vi "Choreo_TrajectoryDifferential_Events.vi"(11 "ChoreoTrajectoryDifferential":T2) -> (3 "events":T1[](array[typedef]))   [LabVIEW 2019, in "ChoreoLib.lvlib"]
doc: "Returns the events in the trajectory.\n\nInputs:\n -- ChoreoTrajectorySwerve - cluster - data cluster for this trajectory \n \nOutputs: \n -- Events - cluster array - the events in the trajectory."
uses:
  ChoreoLib.lvlib
  TypeDef/ChoreoTrajectoryDifferential.ctl
  TypeDef/ChoreoDifferentialSample.ctl
  TypeDef/ChoreoEventMarker.ctl
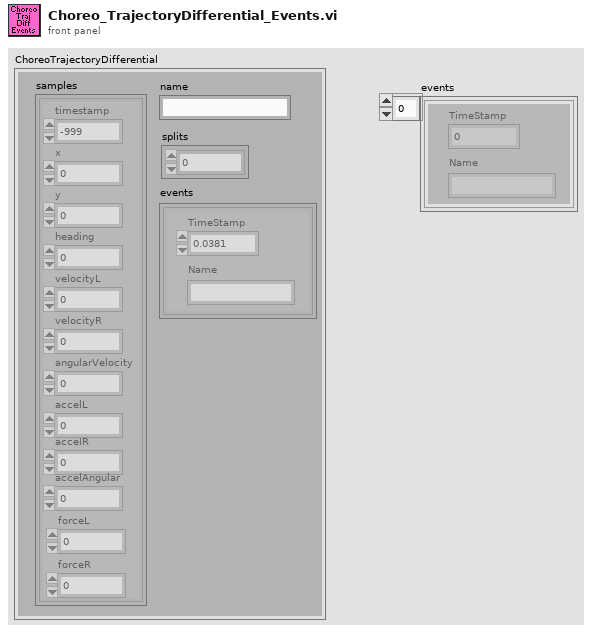
[diagram p1: front panel]
types:
  T1 = typedef "ChoreoLib.lvlib/ChoreoEventMarker.ctl" = cluster{"TimeStamp":dbl, "Name":string}
  T2 = typedef "ChoreoLib.lvlib/ChoreoTrajectoryDifferential.ctl" = cluster{"name":string, "samples":T3[], "splits":i32[], "events":T1[]}
  T3 = typedef "ChoreoLib.lvlib/ChoreoDifferentialSample.ctl" = cluster{"timestamp":dbl, "x":dbl, "y":dbl, "heading":dbl, "velocityL":dbl, "velocityR":dbl, "angularVelocity":dbl, "accelL":dbl, "accelR":dbl, "accelAngular":dbl, "forceL":dbl, "forceR":dbl}
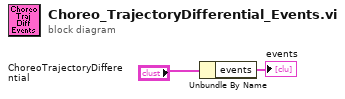
[diagram p0: block diagram]
diagram:
  n1 = Unbundle By Name("ChoreoTrajectoryDifferential") -> ("events"=→"events":T1[])
